vi "Start AI.vi"(0 "reference in":refnum<class "AI.lvclass">, 5 "error in (no error)":errorcluster) -> (14 "reference out":refnum<class "AI.lvclass">, 19 "error out":errorcluster)   [LabVIEW 2017, in "AI.lvclass"]
uses:
  AI.lvclass
  utils/AI_Read.vi
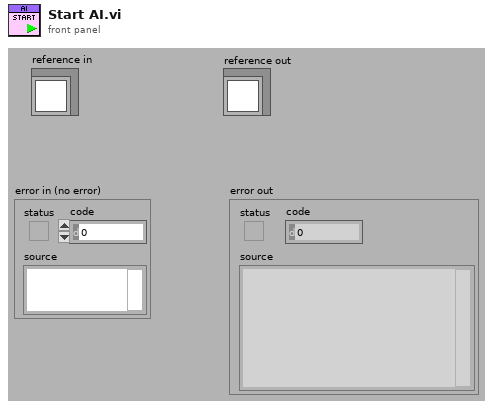
[diagram p1: front panel]
types:
  T1 = typedef "AI.lvclass/ObjectAttributes.ctl" = cluster{"AI Task":refnum<k21>, "AI On/Off Status":bool, "AI Sampling Rate (Samples/Seconds)":u32, "Number of AI Samples Per Channel":i32, "AI Voltage Range":u8, "AI Readings":dbl[][], "Number of AI Modules":i32, "Number of Total AI Channels":i32, "AI Module Names (NI-Max Name)":string[], "Number of Channels Per AI  Module":i32[], "AI VI Reference":refnum<vi>}
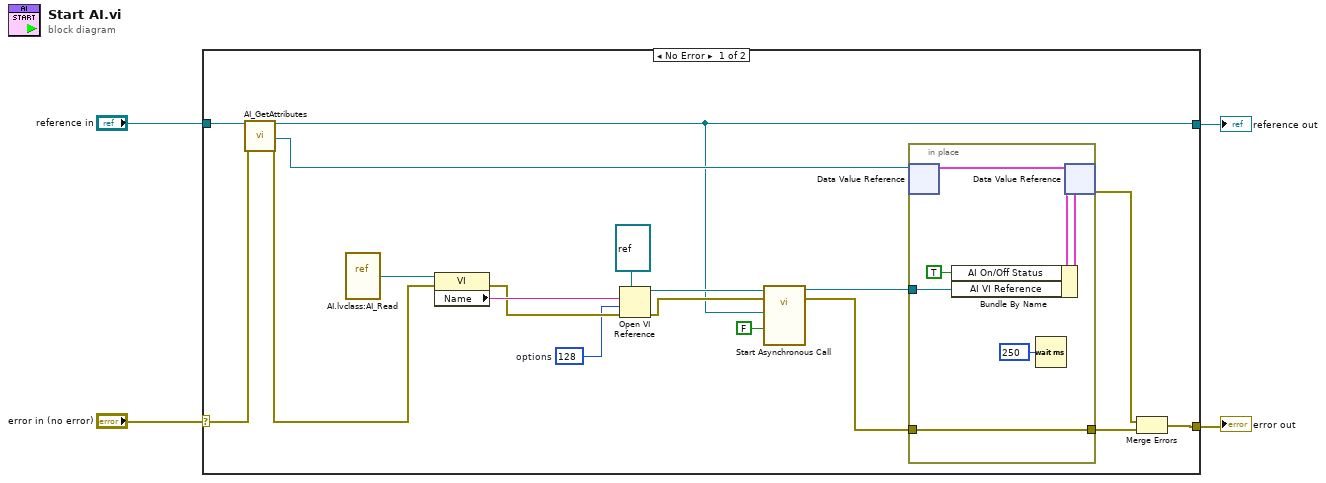
[diagram p0: block diagram]
diagram:
  n1 = case shown="No Error" "error in (no error)" {
    selector: "error in (no error)" -> [w21 w30]
    tunnel: [w19 w30] -> w3
    tunnel: [w7 w29] -> w1
    tunnel: "reference in" -> [w22 w29]
    frame No Error {
      w13 = 128  # options
      n2 = call "AI_GetAttributes.vi"("reference in"=w22, "error in (no error)"=w21) -> ("reference out"=w7:refnum<class "AI.lvclass">, "DataRef"=w18:refnum<data-value>, "error out"=w11:errorcluster)  [unwired: 14 in, 1 out]
      n3 = vi-ref "AI.lvclass:AI_Read.vi"() -> (w15:refnum<vi>)
      n4 = property class="VI"(reference=w15, error in=w11) -> (error out=w14:errorcluster, "Name"=w16:string)  [unwired: 1 out]
      n5 = Open VI Reference(type specifier VI Refnum (for type only)=refnum<vi> refnum, vi path=w16, options=w13, error in (no error)=w14) -> (vi reference=w10:refnum<vi>, error out=w9:errorcluster)  [unwired: 2 in]
      n6 = call-by-ref "Start Asynchronous Call"(reference=w10, error in=w9, "Stop AI"=FALSE ("Stop Temperature"), "reference in"=w7) -> (reference out=w5:refnum<vi>, error out=w6:errorcluster)  [unwired: 8 in, 2 out]
      n7 = in-place {
        in-place-border: w6 -> [w26]
        in-place-border: [w26] -> w17
        in-place-border: w5 -> [w24]
        n8 = in-place-dvr #1(w18) -> (w27:T1)  [unwired: 1 out]
        n9 = Bundle By Name(cluster=w27, "AI On/Off Status"=TRUE, "AI VI Reference"=w24) -> (w28:T1)
        n10 = Wait (ms)(milliseconds to wait=u32 250) -> ()  [unwired: 1 out]
        n11 = in-place-dvr #1(w28) -> (w20:errorcluster)  [unwired: 1 out]
      }
      n12 = Merge Errors(w20, w17) -> (w19:errorcluster)
    }
    frame Error {
    }
  }
  "error out" <- w3
  "reference out" <- w1
